vi "scanallchannels.vi"(0 "VISA resource name in":refnum<visa-resource-name>="81160A", 1 "nm ch":i32[](array[numeric])=[0, 1, 2, 6], 2 "Voltages values":dbl[](array[numeric])=[0.1, 0.5, 1.0], 3 "Init ch value":i32[](array[numeric])=[2500, 2500, 2500, 2500], 4 "base path":path=path "D:/CTA/Data_test/all/backup.lvm", 5 "error in":errorcluster, 6 "Integration Board IP":string="172.16.7.43", 7 "L1 Address":i32=17, 8 "Save test data":bool, 9 "Ch burst":i32=10000, 11 "vclip":i32[](array[numeric])=[0, 0, 0, 0, 0], 13 "Delay":i32) -> (10 "Amp&width":dbl[][](array[numeric]), 12 "VISA resource name out":refnum<visa-resource-name>, 14 "Array":dbl[][](array[numeric]), 15 "L1 min values":i32[](array[numeric])=[180, 378, 779, 1613, 2478, 4286, 5228, 6743], 16 "temperatura":dbl[](array[numeric]), 17 "time":u32[](array[numeric]), 19 "error out":errorcluster)   [LabVIEW 2009]
uses:
  <instrlib>/Agilent 81150/Agilent 81150.lvlib
  <vilib>/Analysis/NI_AALPro.lvlib
  <instrlib>/Agilent 8000 Series/Agilent 8000 Series.lvlib
panel:
  out "read buffer":string
  out "appended array":dbl[](array[numeric])
  out "Pulse Error":dbl caption="Measurement"
  out "Amp Error":dbl caption="Measurement"
  out "Pulse with":dbl caption="Measurement"
  out "Amplitude":dbl caption="Measurement"
  in  "VISA resource name":refnum<visa-resource-name>="Oscilloscope"
  out "Numeric 2":i32
  out "XY Graph 2":cluster{"Y":dbl[], "Y":dbl[]}[](graph)=[{"Y"=[3872.0, 3873.0, 3874.0, 3875.0, 3876.0, 3877.0, 3878.0, 3879.0, 3880.0, 3881.0, 3882.0, 3883.0, 3884.0, 3885.0, 3886.0, 3887.0, 3888.0, 3889.0, 3890.0, 3891.0, 3892.0, 3893.0, 3894.0, 3895.0, 3896.0, 3897.0, 3898.0, 3899.0, 3900.0, 3901.0, 3902.0, 3903.0, 3904.0, 3905.0, 3906.0, 3907.0, 3908.0, 3909.0, 3910.0, 3911.0, 3912.0], "Y"=[7970.0, 8007.0, 7777.0, 7371.0, 7381.0, 7261.0, 7184.0, 6979.0, 6704.0, 6758.0, 6471.0, 6439.0, 6080.0, 6119.0, 5733.0, 5657.0, 5620.0, 5103.0, 5111.0, 4943.0, 4754.0, 4511.0, 4527.0, 4402.0, 4041.0, 3890.0, 3793.0, 3453.0, 3317.0, 3379.0, 3150.0, 3129.0, 2936.0, 2835.0, 2736.0, 2359.0, 2360.0, 2245.0, 2095.0, 2114.0, 1969.0]}]
  out "Data out":string="empty_read_buffer"
  out "Numeric":i32
  out "x .and. y?":bool
  out "XY Graph":cluster{"Y":dbl[], "Y":dbl[]}[](graph)=[{"Y"=[693.0, 694.0, 794.0, 894.0, 994.0, 1094.0, 1194.0, 1294.0, 1394.0, 1494.0, 1594.0, 1694.0, 1794.0, 1894.0, 1994.0, 2094.0, 2194.0, 2294.0, 2394.0, 2494.0, 2594.0, 2694.0, 2794.0, 2894.0, 2994.0, 3094.0, 3194.0, 3294.0, 3394.0, 3494.0, 3594.0, 3694.0, 3794.0, 3894.0, 3994.0, 3795.0, 3805.0, 3815.0, 3825.0, 3806.0, 3807.0, 3808.0, 3809.0, 3810.0, 3811.0, 3812.0, 3813.0, 3814.0, 3815.0, 3816.0, 3817.0, 3818.0, 3819.0, 3820.0, 3821.0, 3822.0, 3823.0, 3824.0, 3825.0, 3826.0, 3827.0, 3828.0, 3829.0, 3830.0, 3831.0, 3832.0, 3833.0, 3834.0, 3835.0, 3836.0, 3837.0, 3838.0, 3839.0, 3840.0, 3841.0, 3842.0, 3843.0, 3844.0, 3845.0, 3846.0, 3847.0, 3848.0, 3849.0, 3850.0, 3851.0, 3852.0, 3853.0, 3854.0, 3855.0, 3856.0, 3857.0, 3858.0, 3859.0, 3860.0, 3861.0, 3862.0, 3863.0, 3864.0, 3865.0, 3866.0, 3867.0, 3868.0, 3869.0, 3870.0, 3871.0, 3872.0, 3873.0, 3874.0, 3875.0, 3876.0, 3877.0, 3878.0, 3879.0, 3880.0, 3881.0, 3882.0, 3883.0, 3884.0, 3885.0, 3886.0, 3887.0, 3888.0, 3889.0, 3890.0, 3891.0, 3892.0, 3893.0, 3894.0, 3895.0, 3896.0, 3897.0, 3898.0, 3899.0, 3900.0, 3901.0, 3902.0, 3903.0, 3904.0, 3905.0, 3906.0, 3907.0, 3908.0, 3909.0, 3910.0, 3911.0, 3912.0, 3913.0, 3914.0, 3915.0, 3916.0, 3917.0, 3918.0, 3919.0, 3920.0, 3921.0, 3922.0, 3923.0, 3924.0, 3925.0, 3926.0, 3927.0, 3928.0, 3929.0, 3930.0, 3931.0, 3932.0, 3933.0, 3934.0, 3935.0, 3936.0, 3937.0, 3938.0, 3939.0, 3940.0, 3941.0, 3942.0, 3943.0, 3944.0], "Y"=[10000.0, 10000.0, 10000.0, 10000.0, 10000.0, 10000.0, 10000.0, 10000.0, 10000.0, 10000.0, 10000.0, 10000.0, 10000.0, 10000.0, 10000.0, 10000.0, 10000.0, 10000.0, 10000.0, 10000.0, 10000.0, 10000.0, 10000.0, 10000.0, 10000.0, 10000.0, 10000.0, 10000.0, 10000.0, 10000.0, 10000.0, 10000.0, 10000.0, 4692.0, 0.0, 9999.0, 10000.0, 9996.0, 9986.0, 9997.0, 10000.0, 10000.0, 9998.0, 9998.0, 9998.0, 9998.0, 10000.0, 9999.0, 9995.0, 9996.0, 9999.0, 9988.0, 9993.0, 9982.0, 9992.0, 9990.0, 9981.0, 9985.0, 9977.0, 9976.0, 9982.0, 9964.0, 9972.0, 9956.0, 9956.0, 9939.0, 9914.0, 9931.0, 9919.0, 9907.0, 9889.0, 9879.0, 9883.0, 9871.0, 9865.0, 9860.0, 9811.0, 9783.0, 9784.0, 9781.0, 9706.0, 9641.0, 9642.0, 9610.0, 9572.0, 9501.0, 9445.0, 9498.0, 9468.0, 9353.0, 9319.0, 9168.0, 9132.0, 9094.0, 8941.0, 9051.0, 8889.0, 8788.0, 8756.0, 8747.0, 8488.0, 8317.0, 8357.0, 8212.0, 8141.0, 7970.0, 8007.0, 7777.0, 7371.0, 7381.0, 7261.0, 7184.0, 6979.0, 6704.0, 6758.0, 6471.0, 6439.0, 6080.0, 6119.0, 5733.0, 5657.0, 5620.0, 5103.0, 5111.0, 4943.0, 4754.0, 4511.0, 4527.0, 4402.0, 4041.0, 3890.0, 3793.0, 3453.0, 3317.0, 3379.0, 3150.0, 3129.0, 2936.0, 2835.0, 2736.0, 2359.0, 2360.0, 2245.0, 2095.0, 2114.0, 1969.0, 1815.0, 1718.0, 1538.0, 1424.0, 1371.0, 1202.0, 1129.0, 1029.0, 1053.0, 949.0, 965.0, 689.0, 672.0, 620.0, 567.0, 617.0, 485.0, 499.0, 361.0, 311.0, 360.0, 274.0, 209.0, 220.0, 244.0, 199.0, 189.0, 199.0, 151.0, 123.0, 116.0, 90.0]}]
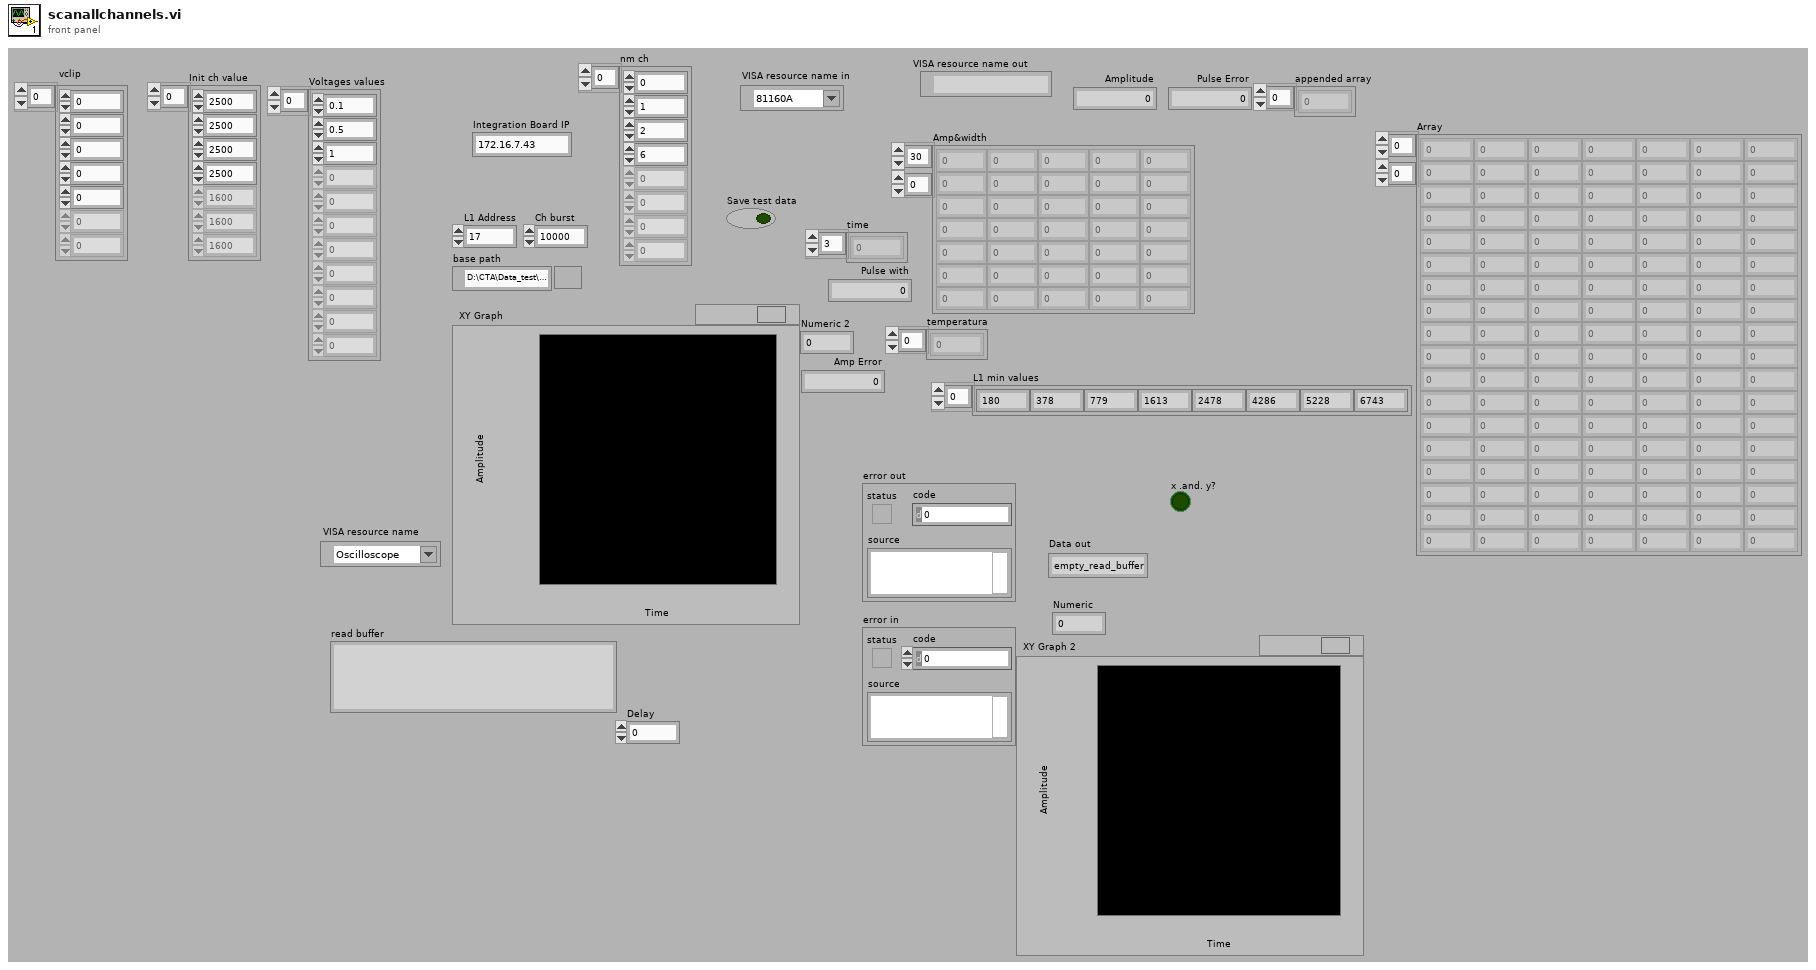
[diagram p1: front panel]
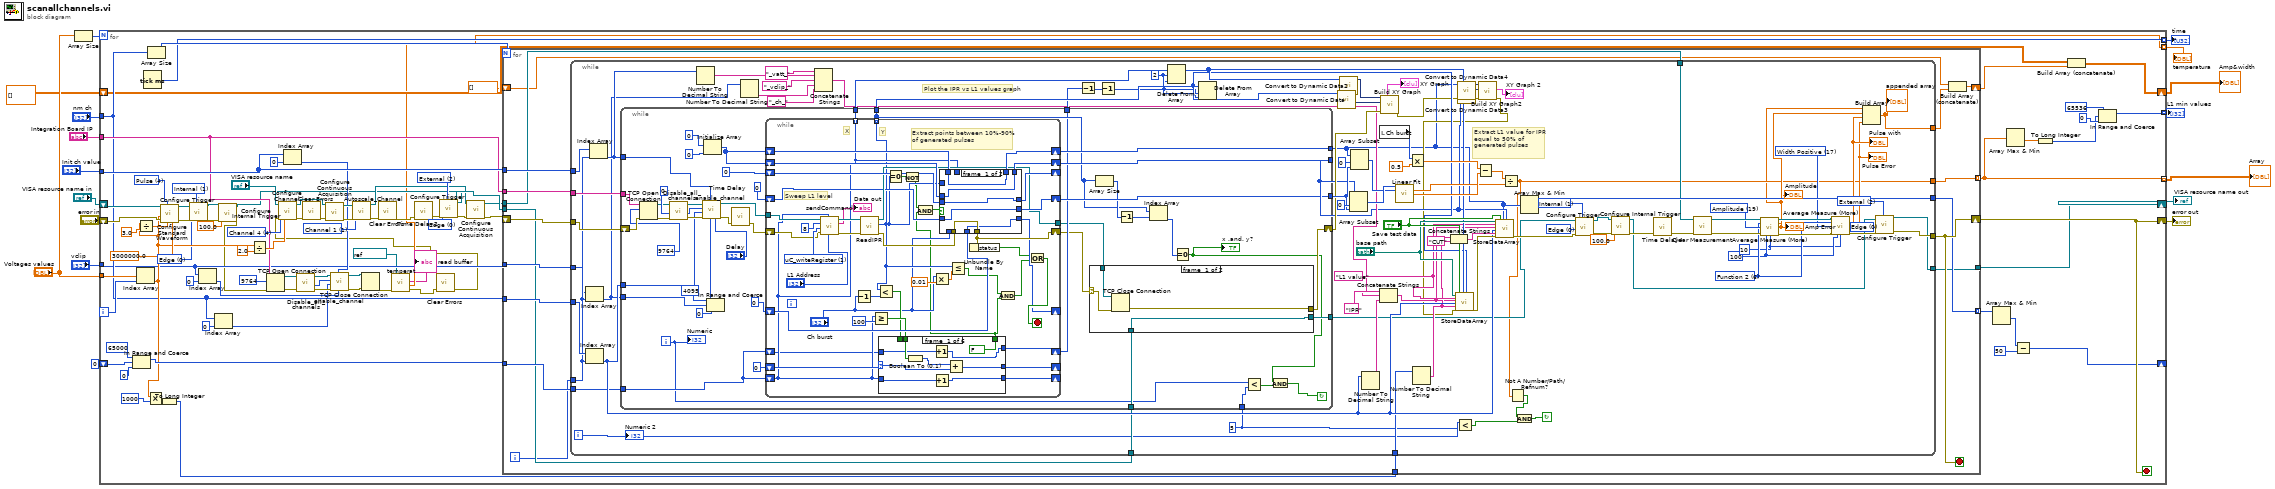
[diagram p0: block diagram]
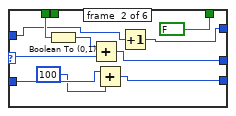
[diagram p2: hidden frame]
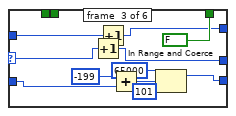
[diagram p3: hidden frame]
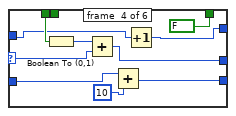
[diagram p4: hidden frame]
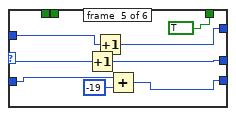
[diagram p5: hidden frame]
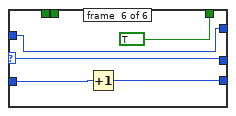
[diagram p6: hidden frame]
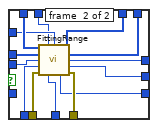
[diagram p7: hidden frame]
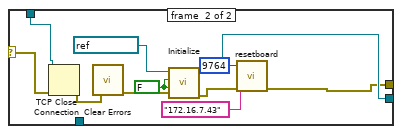
[diagram p8: hidden frame]
diagram:
  n1 = Array Size(array="Voltages values") -> (size(s)=w10:i32)
  n2 = for {
    N: w10 -> [_]
    shift-right: [w92] -> w16
    shift-left: "error in" -> [w91]
    tunnel: [w98] -> w15 mode=indexing
    tunnel: [w93] -> w4 mode=indexing
    tunnel: "Integration Board IP" -> [w47]
    tunnel: "Voltages values" -> [w88]
    tunnel: "Init ch value" -> [w52]
    tunnel: "nm ch" -> [w43]
    tunnel: "vclip" -> [w41]
    shift-right: [w86] -> _
    shift-left: 0 ("State machine") -> [w81]
    shift-right: [w77] -> w6
    shift-left: "VISA resource name in" -> [w94]
    tunnel: [w76] -> w5 mode=indexing
    shift-right: [w35] -> w3
    shift-left: dbl[][] [] -> [w34]
    tunnel: [w21] -> w1 mode=indexing
    i -> [w99]
    stop <- w92 stop-if-true
    w33 = u16 0 items=["Edge", "Level"] ("Trigger Mode (0: Edge)")
    w56 = u16 2 items=["Immediate", "Internal", "External", "Software Trigger Function"] ("Trigger Source (0: Immediate)")
    w57 = u16 0 items=["Edge", "Level"] ("Trigger Mode (0: Edge)")
    w61 = 4 items=["Channel 1"=1, "Channel 2"=2, "Channel 3"=3, "Channel 4"=4] ("Channel (1: Channel 1)")
    w68 = 1 items=["Channel 1"=1, "Channel 2"=2, "Channel 3"=3, "Channel 4"=4, "Function 1"=5, "Function 2"=6, "Function 3"=7, "Function 4"=8, "Memory 1"=9, "Memory 2"=10, "Memory 3"=11, "Memory 4"=12] ("Channel")
    w69 = u16 1 items=["Immediate", "Internal", "External", "Software Trigger Function"] ("Trigger Source (0: Immediate)")
    w103 = u16 4 items=["Sine", "Square", "Ramp Up", "Ramp Down", "Pulse", "Noise", "DC"] ("Waveform (0: Sine)")
    n3 = In Range and Coerce(upper limit=65000, x=w81, lower limit=0) -> (coerced(x)=w80:i32)  [unwired: 1 out]
    n4 = Index Array(array=w88, index=w99) -> (element=w67:dbl)
    n5 = Divide(x=w67, y=3.0) -> (x/y=w101:dbl)
    n6 = Tick Count (ms)() -> (millisecond timer value=w76:u32)
    n7 = Multiply(x=w67, y=1000) -> (x*y=w89:dbl)
    n8 = Array Size(array=w43) -> (size(s)=w95:i32)
    n9 = call <instrlib>:"Configure Standard Waveform.vi"("Frequency (1000.0 Hz)"=3000000.0, "DC Offset (0.0 Volts)"=w101, "Waveform (0: Sine)"=w103, "error in (no error)"=w91, "Amplitude (1.0 Vpp)"=w67, "VISA resource name"=w94) -> ("error out"=w74:errorcluster, "VISA resource name out"=w75:refnum<visa-resource-name>)  [unwired: 4 in]
    n10 = To Long Integer(number=w89) -> (32bit integer=w87:i32)
    n11 = call <instrlib>:"Configure Trigger.vi"("Trigger Source (0: Immediate)"=w69, "error in (no error)"=w74, "Trigger Mode (0: Edge)"=w33, "VISA resource name"=w75) -> ("error out"=w32:errorcluster, "VISA resource name out"=w30:refnum<visa-resource-name>)  [unwired: 6 in]
    n12 = Index Array(array=w41, index=0) -> (element=w27:i32)
    n13 = Index Array(array=w43, index=0) -> (element=w26:i32)
    n14 = call <instrlib>:"Configure Internal Trigger.vi"("error in (no error)"=w32, "Frequency (100000.0 Hz)"=100.0, "VISA resource name"=w30) -> ("error out"=w31:errorcluster, "VISA resource name out"=w29:refnum<visa-resource-name>)  [unwired: 7 in]
    n15 = Divide(x=w67, y=2.0) -> (x/y=w60:dbl)
    n16 = TCP Open Connection(address=w47, remote port or service name=u16 9764, error in (no error)=w31) -> (connection ID=w46:refnum<k5>, error out=w48:errorcluster)  [unwired: 2 in]
    n17 = Index Array(array=w52, index=0) -> (element=w50:i32)
    n18 = call "Disable_all_channels.vi"("error in"=w48, "connection ID"=w46) -> ("error out"=w49:errorcluster, "id_out"=w40:i32, "connection ID out"=w45:refnum<k5>)  [unwired: 7 in]
    n19 = call "enable_channel.vi"("V clip"=w27, "V att"=w50, "error in"=w49, "Channel"=w26, "id_in"=w40, "connection ID"=w45) -> ("error out"=w38:errorcluster, "connection ID out"=w39:refnum<k5>)  [unwired: 3 in, 1 out]
    n20 = TCP Close Connection(connection ID=w39, error in (no error)=w38) -> (error out=w23:errorcluster)  [unwired: 1 in, 1 out]
    n21 = call "temperat.vi"("error in (no error)"=w23, "VISA resource name"=refnum<visa-resource-name> "COM1") -> ("error out"=w20:errorcluster, "number"=w21:dbl, "read buffer"=→"read buffer":string)  [unwired: 2 in, 1 out]
    n22 = call <vilib>:"Clear Errors.vi"("error in (no error)"=w20) -> ("error out"=w19:errorcluster)  [unwired: 6 in]
    n23 = call <instrlib>:"Configure Channel.vi"("VISA resource name"="VISA resource name", "Channel (1: Channel 1)"=w61, "error in (no error)"=w19, "Vertical Range (2.0 V)"=w60) -> ("VISA resource name out"=w62:refnum<visa-resource-name>, "error out"=w65:errorcluster)  [unwired: 10 in]
    n24 = call <vilib>:"Clear Errors.vi"("error in (no error)"=w65) -> ("error out"=w64:errorcluster)  [unwired: 6 in]
    n25 = call <instrlib>:"Configure Continuous Acquisition.vi"("error in (no error)"=w64, "VISA resource name"=w62) -> ("error out"=w73:errorcluster, "VISA resource name out"=w71:refnum<visa-resource-name>)  [unwired: 8 in]
    n26 = call "Autoscale_Channel.vi"("error in"=w73, "Channel"=w68, "VISA resource name"=w71) -> ("error out"=w72:errorcluster, "VISA resource name out"=w53:refnum<visa-resource-name>)  [unwired: 5 in, 2 out]
    n27 = call <vilib>:"Clear Errors.vi"("error in (no error)"=w72) -> ("error out"=w70:errorcluster)  [unwired: 6 in]
    n28 = call "Time Delay2"("error in (no error)"=w70) -> ("error out"=w59:errorcluster)  [unwired: 10 in]
    n29 = call <instrlib>:"Configure Trigger.vi"("Trigger Source (0: Immediate)"=w56, "error in (no error)"=w59, "Trigger Mode (0: Edge)"=w57, "VISA resource name"=w29) -> ("error out"=w54:errorcluster, "VISA resource name out"=w58:refnum<visa-resource-name>)  [unwired: 6 in]
    n30 = call <instrlib>:"Configure Continuous Acquisition.vi"("error in (no error)"=w54, "VISA resource name"=w53) -> ("error out"=w55:errorcluster, "VISA resource name out"=w36:refnum<visa-resource-name>)  [unwired: 8 in]
    n31 = for {
      N: w95 -> [_]
      tunnel: [w121] -> w93 mode=indexing
      shift-right: [w116] -> w92
      shift-left: w55 -> [w119]
      tunnel: w43 -> [w120]
      tunnel: w47 -> [w118]
      tunnel: w52 -> [w117]
      tunnel: w41 -> [w115]
      tunnel: w87 -> [w114]
      tunnel: w80 -> [w113]
      tunnel: [w112] -> w83 mode=indexing
      tunnel: w58 -> [w110]
      tunnel: [w111] -> w77
      tunnel: w36 -> [w108]
      shift-right: [w107] -> w24
      shift-left: dbl[] [] -> [w105]
      i -> [w109]
      stop <- w116 stop-if-true
      n32 = while {
        tunnel: [w135] -> w121
        tunnel: w120 -> [w203]
        tunnel: w119 -> [w202]
        tunnel: w118 -> [w201]
        tunnel: w117 -> [w197]
        tunnel: [w133] -> w116
        tunnel: w109 -> [w192]
        tunnel: w115 -> [w191]
        tunnel: w114 -> [w180]
        tunnel: w113 -> [w161]
        tunnel: [w159] -> w112
        tunnel: [w131] -> w111
        tunnel: w110 -> [w158]
        tunnel: w108 -> [w146]
        tunnel: [w134] -> w106
        i -> [w154]
        stop <- w156 continue-if-true
        w129 = u16 2 items=["Immediate", "Internal", "External", "Software Trigger Function"] ("Trigger Source (0: Immediate)")
        w130 = u16 0 items=["Edge", "Level"] ("Trigger Mode (0: Edge)")
        w139 = u32 10 ("Max Errors")
        w140 = u32 100 ("Averages")
        w141 = 17 items=["Rise Time", "Fall Time", "Frequency", "Period", "Voltage RMS(AC)", "Voltage RMS(DC)", "Voltage RMS (AC,cycle)", "Voltage RMS (DC,cycle)", "Voltage Max", "Voltage Min", "Voltage Middle", "Voltage Vpp", "Voltage High", "Voltage Low", "Voltage Average", "Voltage Average (cycle)", "Width Negative", "Width Positive", "Duty Cycle Positive", "Amplitude", "Overshoot", "Preshoot", "Voltage Base", "Voltage Upper", "Time Max", "Time Min", "Color Grade Crossing", "Color Grade Eye Width", "Color Grade Eye Height", "Color Grade Eye Q-Factory", "Color Grade Eye Duty Cycle Distortion(Percent)", "Color Grade Eye Duty Cycle Distortion(Time)", "Color Grade Eye Jitter(PP)", "Color Grade Eye Width(RMS)", "Cycle-cycle Duty Jitter(Rising)", "Cycle-cycle Duty Jitter(Falling)", "Cycle-cycle Jitter(Rising)", "Cycle-cycle Jitter(Falling)", "Cycle-cycle - Width", "Cycle-cycle + Width", "Date Rate", "Unit Interval", "FFT Delta Frequency", "FFT Delta Magnitude", "FFT Frequency", "FFT Magnitude", "Slew Rate", "Area (Entire Display)", "Area(Single Cycle)", "Duty Cycle (Rising)", "Duty Cycle (Falling)"] ("Measurement Function (0: Rise Time)")
        w145 = 19 items=["Rise Time", "Fall Time", "Frequency", "Period", "Voltage RMS(AC)", "Voltage RMS(DC)", "Voltage RMS (AC,cycle)", "Voltage RMS (DC,cycle)", "Voltage Max", "Voltage Min", "Voltage Middle", "Voltage Vpp", "Voltage High", "Voltage Low", "Voltage Average", "Voltage Average (cycle)", "Width Negative", "Width Positive", "Duty Cycle Positive", "Amplitude", "Overshoot", "Preshoot", "Voltage Base", "Voltage Upper", "Time Max", "Time Min", "Color Grade Crossing", "Color Grade Eye Width", "Color Grade Eye Height", "Color Grade Eye Q-Factory", "Color Grade Eye Duty Cycle Distortion(Percent)", "Color Grade Eye Duty Cycle Distortion(Time)", "Color Grade Eye Jitter(PP)", "Color Grade Eye Width(RMS)", "Cycle-cycle Duty Jitter(Rising)", "Cycle-cycle Duty Jitter(Falling)", "Cycle-cycle Jitter(Rising)", "Cycle-cycle Jitter(Falling)", "Cycle-cycle - Width", "Cycle-cycle + Width", "Date Rate", "Unit Interval", "FFT Delta Frequency", "FFT Delta Magnitude", "FFT Frequency", "FFT Magnitude", "Slew Rate", "Area (Entire Display)", "Area(Single Cycle)", "Duty Cycle (Rising)", "Duty Cycle (Falling)"] ("Measurement Function (0: Rise Time)")
        w142 = 6 items=["Channel 1"=1, "Channel 2"=2, "Channel 3"=3, "Channel 4"=4, "Function 1"=5, "Function 2"=6, "Function 3"=7, "Function 4"=8, "Memory 1"=9, "Memory 2"=10, "Memory 3"=11, "Memory 4"=12] ("Channel (1: Channel 1)")
        w149 = u16 0 items=["Edge", "Level"] ("Trigger Mode (0: Edge)")
        w150 = u16 1 items=["Immediate", "Internal", "External", "Software Trigger Function"] ("Trigger Source (0: Immediate)")
        w153 = 5 ("y")
        w185 = 2 ("length")
        w182 = "L1 value" ("X Signal Name")
        # "Extract L1 value for IPR equal to 50% of generated pulses"
        # "Plot the IPR vs L1 values graph"
        n33 = Index Array(array=w203, index=w192) -> (element=w181:i32)
        n34 = Index Array(array=w191, index=w192) -> (element=w177:i32)
        n35 = Index Array(array=w197, index=w192) -> (element=w178:i32)
        n36 = while {
          tunnel: [w258] -> w160
          tunnel: [w242] -> w166
          tunnel: [w257] -> w211
          tunnel: [w237] -> w188
          tunnel: [w239] -> w190
          tunnel: w181 -> [w249]
          tunnel: w201 -> [w245]
          shift-right: [w223] -> w194
          shift-left: w202 -> [w248]
          tunnel: w178 -> [w236]
          tunnel: w177 -> [w235]
          tunnel: [w231] -> w186
          tunnel: w161 -> [w230]
          tunnel: [w228] -> w147
          tunnel: w158 -> [w227]
          tunnel: w153 -> [w217]
          i -> [w218]
          stop <- w221 continue-if-true
          n37 = TCP Open Connection(address=w245, remote port or service name=u16 9764, error in (no error)=w248) -> (connection ID=w246:refnum<k5>, error out=w247:errorcluster)  [unwired: 2 in]
          n38 = call "Disable_all_channels.vi"("error in"=w247, "id_in"=0, "connection ID"=w246) -> ("error out"=w254:errorcluster, "id_out"=w251:i32, "connection ID out"=w253:refnum<k5>)  [unwired: 6 in]
          n39 = Initialize Array(0 ("element"), 0 ("dimension size")) -> (w260:i32[])
          n40 = In Range and Coerce(upper limit=4095, x=w235, lower limit=0) -> (coerced(x)=w232:i32)  [unwired: 1 out]
          n41 = call "enable_channel.vi"("Delay"="Delay", "V clip"=w232, "V att"=w236, "error in"=w254, "Channel"=w249, "id_in"=w251, "connection ID"=w253) -> ("error out"=w226:errorcluster, "connection ID out"=w252:refnum<k5>)  [unwired: 2 in, 1 out]
          n42 = call "Time Delay"("error in (no error)"=w226) -> ("error out"=w225:errorcluster)  [unwired: 10 in]
          n43 = while {
            tunnel: [w268] -> w237 mode=indexing
            tunnel: [w276] -> w239 mode=indexing
            shift-right: [w303] -> w258
            shift-left: w260 -> [w301]
            shift-right: [w302] -> w242
            shift-left: w260 -> [w300]
            shift-right: [w296] -> w224
            shift-left: w225 -> [w285]
            shift-right: [w298] -> _
            shift-left: 0 ("Array Pointer out") -> [w299]
            tunnel: w252 -> [w286]
            tunnel: [w287] -> w222
            shift-right: [w297] -> w257
            shift-left: 0 ("N_Array Elements") -> [w284]
            shift-right: [w282] -> _
            shift-left: 0 ("State machine") -> [w283]
            shift-right: [w278] -> _
            shift-left: 0 -> [w280]
            shift-right: [w277] -> _
            shift-left: w230 -> [w276]
            shift-right: [w274] -> w231
            shift-left: w230 -> [w273]
            stop <- w295 stop-if-true
            w293 = u16 1 items=["sendCommand"=9, "FPGA_writeRegister"=3, "FPGA_readRegister"=2, "uC_writeRegister"=1, "uC_readRegister"=0] ("Action")
            # "Extract points between 10%-90% of generated pulses"
            # "Sweep L1 level"
            # "Y"
            # "X"
            n44 = call "sendCommand.vi"("Address"="L1 Address", "Data"=w276, "error in"=w285, "Action"=w293, "id_in"=8 ("id"), "connection ID"=w286) -> ("error out"=w292:errorcluster, "Data out"=→"Data out":string, "connection ID out"=w291:refnum<k5>)  [unwired: 1 in, 2 out]
            n45 = Decrement(x="Ch burst") -> (x-1=w272:i32)
            n46 = call "ReadIPR.vi"("error in"=w292, "connection ID"=w291) -> ("error out"=w290:errorcluster, "IPR value"=w268:i32, "connection ID out"=w287:refnum<k5>)  [unwired: 5 in, 2 out]
            n47 = Greater Or Equal?(x=w276, y=100) -> (x >= y?=w279:bool)
            n48 = Less?(x=w268, y=w272) -> (x < y?=w275:bool)
            n49 = case shown="0, Default" w280 {
              selector: w280 -> [w312 w322 w335 w340 w349 w356]
              tunnel: w279 -> [w314 _ _ _ _ _]
              tunnel: [w311 w321 w331 w338 w348 w356] -> w278
              tunnel: [w309 w318 w327 w343 w351 w357] -> w277
              tunnel: w276 -> [w310 w320 w334 w344 w352 w358]
              tunnel: w275 -> [_ w324 _ w341 _ _]
              tunnel: [FALSE FALSE FALSE FALSE TRUE TRUE] -> w266
              tunnel: [w307 w316 w330 w337 w347 w354] -> w274
              tunnel: w273 -> [w306 w315 w329 w336 w350 w354]
              frame #0 {
                n50 = Boolean To (0,1)(Boolean=w314) -> (0, 1=w313:i16)
                n51 = Increment(x=w306) -> (x+1=w307:i32)
                n52 = Increment(x=w310) -> (x+1=w309:i32)
                n53 = Add(x=w313, y=w312) -> (x+y=w311:i32)
              }
              frame #1 {
                n54 = Boolean To (0,1)(Boolean=w324) -> (0, 1=w323:i16)
                n55 = Add(x=w323, y=w322) -> (x+y=w321:i32)
                n56 = Add(x=w320, y=100) -> (x+y=w318:i32)
                n57 = Increment(x=w315) -> (x+1=w316:i32)
              }
              frame #2 {
                n58 = Increment(x=w335) -> (x+1=w331:i32)
                n59 = Increment(x=w329) -> (x+1=w330:i32)
                n60 = Add(x=-199, y=w334) -> (x+y=w328:i32)
                n61 = In Range and Coerce(upper limit=65000, x=w328, lower limit=101) -> (coerced(x)=w327:i32)  [unwired: 1 out]
              }
              frame #3 {
                n62 = Boolean To (0,1)(Boolean=w341) -> (0, 1=w339:i16)
                n63 = Add(x=w339, y=w340) -> (x+y=w338:i32)
                n64 = Add(x=w344, y=10) -> (x+y=w343:i32)
                n65 = Increment(x=w336) -> (x+1=w337:i32)
              }
              frame #4 {
                n66 = Increment(x=w349) -> (x+1=w348:i32)
                n67 = Increment(x=w350) -> (x+1=w347:i32)
                n68 = Add(x=w352, y=-19 ("x")) -> (x+y=w351:i32)
              }
              frame #5 {
                n69 = Increment(x=w358) -> (x+1=w357:i32)
              }
            }
            n70 = Equal To 0?(x=w268) -> (x = 0?=w264:bool)
            n71 = Not(x=w264) -> (.not. x?=w263:bool)
            n72 = And(x=w263, y=w266) -> (x .and. y?=w265:bool)
            n73 = Multiply(x="Ch burst", y=0.01) -> (x*y=w304:dbl)
            n74 = case shown="False" w265 {
              tunnel: [w364 w378] -> w303
              tunnel: [w363 w377] -> w302
              tunnel: w301 -> [w364 w376]
              tunnel: w300 -> [w363 w375]
              tunnel: w299 -> [w361 w374]
              tunnel: [w361 w373] -> w298
              tunnel: [w360 w372] -> w297
              tunnel: "Ch burst" -> [_ w371]
              tunnel: [w362 w370] -> w296
              tunnel: w290 -> [w362 w369]
              tunnel: w268 -> [_ w368]
              tunnel: w276 -> [_ w367]
              tunnel: w284 -> [w360 _]
              tunnel: w283 -> [w359 w366]
              tunnel: [w359 w365] -> w282
              frame #0 {
              }
              frame #1 {
                n75 = call "FittingRange.vi"("Array in (X)"=w376, "L0 DAC"=w367, "IPR"=w368, "Array in (Y)"=w375, "Array Pointer in"=w374, "Cycles Burst"=w371, "error in"=w369, "State machine"=w366) -> ("Array out (X)"=w378:i32[], "Array out (Y)"=w377:i32[], "Array Pointer out"=w373:i32, "N_Array Elements"=w372:i32, "State machine"=w365:i32, "error out"=w370:errorcluster)  [unwired: 2 in]
              }
            }
            n76 = Less Or Equal?(x=w268, y=w304) -> (x <= y?=w271:bool)
            n77 = Unbundle By Name(w296) -> ("status"=w269:bool)
            n78 = And(x=w271, y=w266) -> (x .and. y?=w270:bool)
            n79 = Or(x=w269, y=w270) -> (x .or. y?=w295:bool)
          }
          n80 = case shown="Error" w224 {
            selector: w224 -> [w382 w393]
            tunnel: [w379 w383] -> w223
            tunnel: [w381 w389] -> w228
            tunnel: w227 -> [w381 _]
            tunnel: w222 -> [w380 w387]
            frame #0 {
              n81 = TCP Close Connection(connection ID=w380, error in (no error)=w382) -> (error out=w379:errorcluster)  [unwired: 1 in, 1 out]
            }
            frame #1 {
              w391 = FALSE ("Reset (True)")
              n82 = TCP Close Connection(connection ID=w387, error in (no error)=w393) -> (error out=w388:errorcluster)  [unwired: 1 in, 1 out]
              n83 = call <vilib>:"Clear Errors.vi"("error in (no error)"=w388) -> ("error out"=w392:errorcluster)  [unwired: 6 in]
              n84 = call <instrlib>:"Initialize.vi"("error in (no error)"=w392, "Reset (True)"=w391, "ID Query (True)"=w391, "VISA resource name"=refnum<visa-resource-name> "81160A") -> ("error out"=w386:errorcluster, "VISA resource name out"=w389:refnum<visa-resource-name>)  [unwired: 6 in]
              n85 = call "resetboard.vi"("error in (no error)"=w386, "address"="172.16.7.43", "remote port or service name"=u16 9764) -> ("error out"=w383:errorcluster)  [unwired: 7 in, 1 out]
            }
          }
          n86 = Array Size(array=w237) -> (size(s)=w240:i32)
          n87 = Decrement(x=w240) -> (x-1=w241:i32)
          n88 = Index Array(array=w237, index=w241) -> (element=w238:i32)
          n89 = Equal To 0?(x=w238) -> (x = 0?=w220:bool)
          "x .and. y?" <- w220
          n90 = Less?(x=w218, y=w217) -> (x < y?=w219:bool)
          n91 = And(x=w220, y=w219) -> (x .and. y?=w221:bool)
          "Numeric" <- w218
        }
        n92 = Number To Decimal String(number=w178) -> (decimal integer string=w176:string)  [unwired: 1 in]
        n93 = Number To Decimal String(number=w177) -> (decimal integer string=w175:string)  [unwired: 1 in]
        n94 = Concatenate Strings("_vatt_" ("string"), w176, "_vclip_" ("string"), w175, "_ch_" ("string")) -> (w169:string)
        n95 = Decrement(x=w186) -> (x-1=w183:i32)
        n96 = Decrement(x=w183) -> (x-1=w184:i32)
        n97 = Delete From Array(array=w190, length=w185, index=w184) -> (array with subset deleted=w189:i32[])  [unwired: 1 out]
        n98 = Delete From Array(array=w188, length=w185, index=w184) -> (array with subset deleted=w187:i32[])  [unwired: 1 out]
        n99 = call "Convert to Dynamic Data"("Array"=w187) -> ("Dynamic Data Type"=w215:dynamicdata)  [unwired: 3 in]
        n100 = call "Convert to Dynamic Data2"("Array"=w189) -> ("Dynamic Data Type"=w214:dynamicdata)  [unwired: 3 in]
        n101 = Array Subset(array=w166, index=0, length=w211) -> (w210:i32[])
        n102 = Array Subset(array=w160, index=0, length=w211) -> (w209:i32[])
        n103 = Number To Decimal String(number=w181) -> (decimal integer string=w168:string)  [unwired: 1 in]
        n104 = Concatenate Strings("IPR" ("Y Signal Name"), w169, w168) -> (w170:string)
        n105 = local read "Ch burst"() -> (w196:i32)
        n106 = call "Build XY Graph"("error in (no error)"=w194, "Y Input"=w215, "X Input"=w214) -> ("error out"=w164:errorcluster, "XY Graph"=→"XY Graph":cluster{"Y":dbl[], "Y":dbl[]}[])  [unwired: 7 in]
        n107 = call <vilib>:"Linear Fit.vi"("Y"=w210, "X"=w209) -> ("slope"=w204:dbl, "intercept"=w206:dbl)  [unwired: 9 in, 3 out]
        n108 = Multiply(x=w196, y=0.5) -> (x*y=w207:dbl)
        n109 = Number To Decimal String(number=w180) -> (decimal integer string=w179:string)  [unwired: 1 in]
        n110 = Concatenate Strings(w179, "CUT" ("string")) -> (w199:string)
        n111 = Less?(x=w154, y=w153) -> (x < y?=w155:bool)
        n112 = call "Convert to Dynamic Data3"("Array"=w160) -> ("Dynamic Data Type"=w167:dynamicdata)  [unwired: 3 in]
        n113 = call "Convert to Dynamic Data4"("Array"=w166) -> ("Dynamic Data Type"=w165:dynamicdata)  [unwired: 3 in]
        n114 = Subtract(x=w207, y=w206) -> (x-y=w205:dbl)
        n115 = call "Build XY Graph2"("error in (no error)"=w164, "Y Input"=w165, "X Input"=w167) -> ("error out"=w163:errorcluster, "XY Graph"=→"XY Graph 2":cluster{"Y":dbl[], "Y":dbl[]}[])  [unwired: 7 in]
        n116 = call "StoreDataArray.vi"("Base path"="base path", "X Signal Name"=w182, "Y Signal Name"=w170, "Channel number"=w181, "Si"=w179, "error in"=w163, "Save test data"="Save test data", "X Array"=w189, "Y Array"=w187) -> ("error out"=w200:errorcluster)  [unwired: 10 in]
        n117 = call "StoreDataArray.vi"("Base path"="base path", "X Signal Name"=w182, "Y Signal Name"=w170, "Channel number"=w181, "Si"=w199, "error in"=w200, "Save test data"="Save test data", "X Array"=w160, "Y Array"=w166) -> ("error out"=w151:errorcluster)  [unwired: 10 in]
        n118 = Divide(x=w205, y=w204) -> (x/y=w135:dbl)
        n119 = Not A Number/Path/Refnum?(number/path/refnum=w135) -> (NaN/Path/Refnum?=w157:bool)
        n120 = And(x=w157, y=w155) -> (x .and. y?=w156:bool)
        n121 = Array Max & Min(array=w160) -> (max value=w159:i32)  [unwired: 3 out]
        n122 = call <instrlib>:"Configure Trigger.vi"("Trigger Source (0: Immediate)"=w150, "error in (no error)"=w151, "Trigger Mode (0: Edge)"=w149, "VISA resource name"=w147) -> ("error out"=w127:errorcluster, "VISA resource name out"=w124:refnum<visa-resource-name>)  [unwired: 6 in]
        n123 = call <instrlib>:"Configure Internal Trigger.vi"("error in (no error)"=w127, "Frequency (100000.0 Hz)"=100.0, "VISA resource name"=w124) -> ("error out"=w126:errorcluster, "VISA resource name out"=w125:refnum<visa-resource-name>)  [unwired: 7 in]
        n124 = call "Time Delay4"("error in (no error)"=w126) -> ("error out"=w128:errorcluster)  [unwired: 10 in]
        n125 = call <instrlib>:"Clear Measurement.vi"("error in (no error)"=w128, "VISA resource name"=w146) -> ("error out"=w152:errorcluster, "VISA resource name out"=w148:refnum<visa-resource-name>)  [unwired: 8 in]
        n126 = call "Average Measure (More).vi"("VISA resource name"=w148, "Channel (1: Channel 1)"=w142, "Measurement Function (0: Rise Time)"=w145, "error in (no error)"=w152, "Averages"=w140, "Max Errors"=w139) -> ("VISA resource name out"=w144:refnum<visa-resource-name>, "Measure Average"=w122:dbl, "Measure Error"=w138:dbl, "error out"=w143:errorcluster)  [unwired: 6 in]
        "Amplitude" <- w122
        "Amp Error" <- w138
        n127 = call "Average Measure (More).vi"("VISA resource name"=w144, "Channel (1: Channel 1)"=w142, "Measurement Function (0: Rise Time)"=w141, "error in (no error)"=w143, "Averages"=w140, "Max Errors"=w139) -> ("Measure Average"=w137:dbl, "Measure Error"=w136:dbl, "error out"=w132:errorcluster)  [unwired: 6 in, 1 out]
        "Pulse with" <- w137
        "Pulse Error" <- w136
        n128 = Build Array(w122, w138, w137, w136) -> (w134:dbl[])
        "appended array" <- w134
        n129 = call <instrlib>:"Configure Trigger.vi"("Trigger Source (0: Immediate)"=w129, "error in (no error)"=w132, "Trigger Mode (0: Edge)"=w130, "VISA resource name"=w125) -> ("error out"=w133:errorcluster, "VISA resource name out"=w131:refnum<visa-resource-name>)  [unwired: 6 in]
        "Numeric 2" <- w154
      }
      n130 = Build Array (concatenate)(w105, w106) -> (w107:dbl[])
    }
    n131 = Array Max & Min(array=w83) -> (min value=w82:i32)  [unwired: 3 out]
    n132 = Array Max & Min(array=w93) -> (min value=w100:dbl)  [unwired: 3 out]
    n133 = Subtract(x=w82, y=50) -> (x-y=w86:i32)
    n134 = To Long Integer(number=w100) -> (32bit integer=w84:i32)
    n135 = Build Array (concatenate)(w34, w24) -> (w35:dbl[][])
    n136 = In Range and Coerce(upper limit=65536, x=w84, lower limit=0) -> (coerced(x)=w98:i32)  [unwired: 1 out]
  }
  "L1 min values" <- w15
  "error out" <- w16
  "VISA resource name out" <- w6
  "time" <- w5
  "Array" <- w4
  "Amp&width" <- w3
  "temperatura" <- w1
